vi "数据查询_仪器日志.vi"() -> ()   [LabVIEW 2016]
uses:
  <vilib>/Utility/miscctls.llb/LVPointTypeDef.ctl
  <vilib>/Utility/miscctls.llb/LVRowAndColumnUnsignedTypeDef.ctl
  <userlib>/_OpenG.lib/array/array.llb/Sort 2D Array (String)__ogtk.vi
panel:
  in  "页":i32 format="第%.0f页"
  in  "每页条数":i32=20
  in  "向后按钮":bool
  in  "向前按钮":bool
  in  "下拉列表":string(xcontrol)
  in  "导出":bool
  in  "查询":bool
  out "数据表":string[][](table)
  in  "结束日期":string="2050/01/01"
  in  "起始日期":string="2010/01/01"
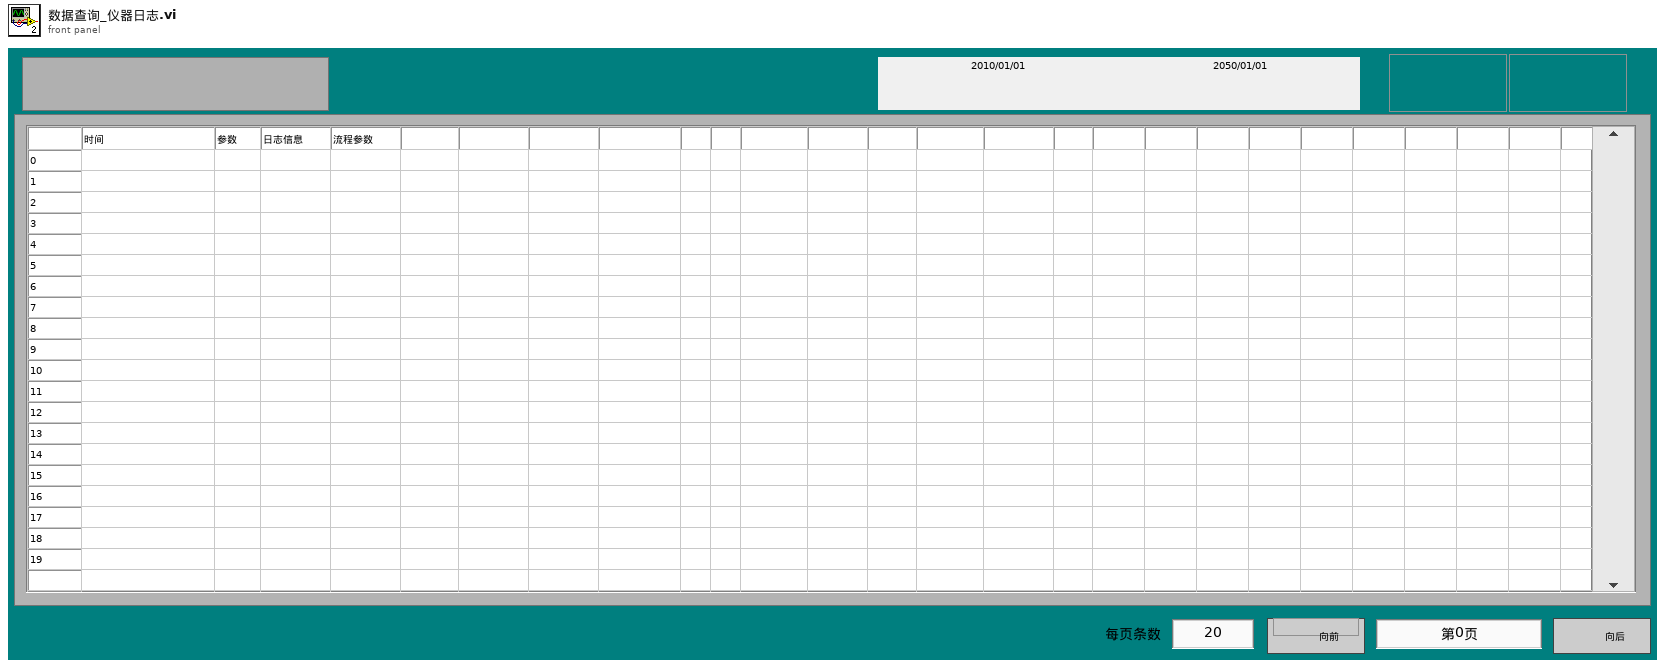
[diagram p1: front panel]
types:
  T1 = enum8{"Enabled", "Disabled", "Disabled and Grayed Out"}
  T2 = typedef "LVRowAndColumnUnsignedTypeDef.ctl" = cluster{"Row":u32, "Column":u32}
  T3 = typedef "LVPointTypeDef.ctl" = cluster{"Horizontal":i16, "Vertical":i16}
  T4 = typedef "LVDateTimeRec.ctl" = cluster{"秒数的小数部分":dbl, "秒":i32, "分":i32, "时":i32, "日":i32, "月":i32, "年":i32, "天数（周）":i32, "天数（年）":i32, "DST":i32}
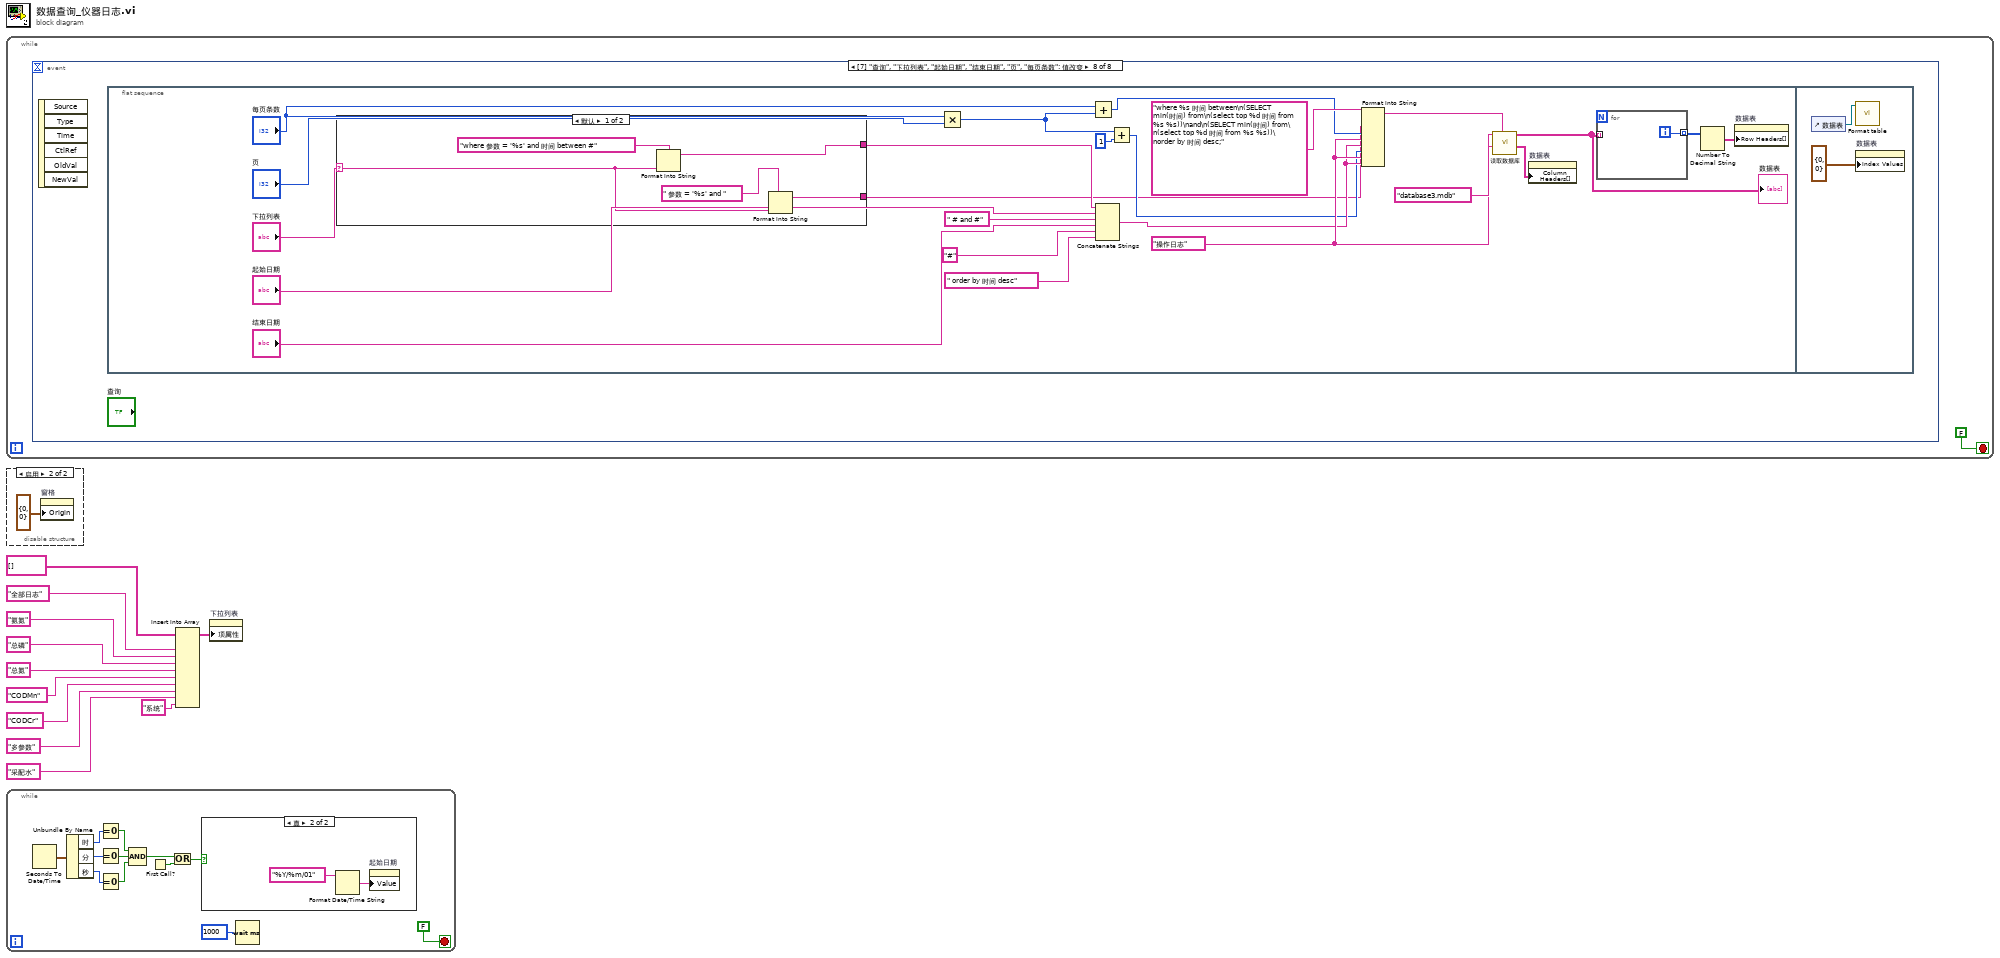
[diagram p0: block diagram]
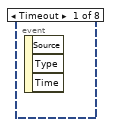
[diagram p3: hidden frame]
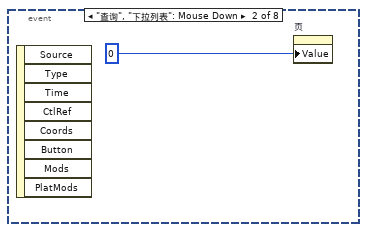
[diagram p4: hidden frame]
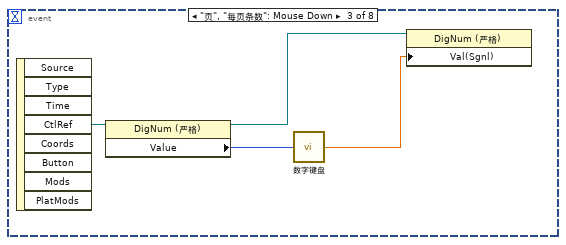
[diagram p5: hidden frame]
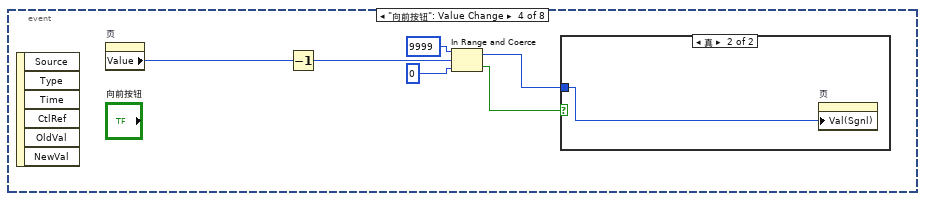
[diagram p6: hidden frame]
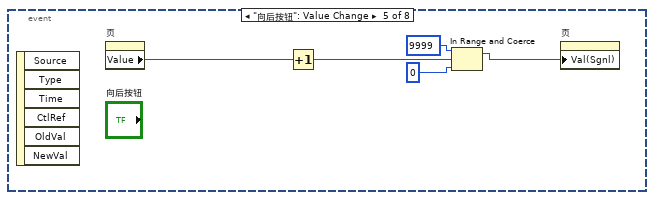
[diagram p8: hidden frame]
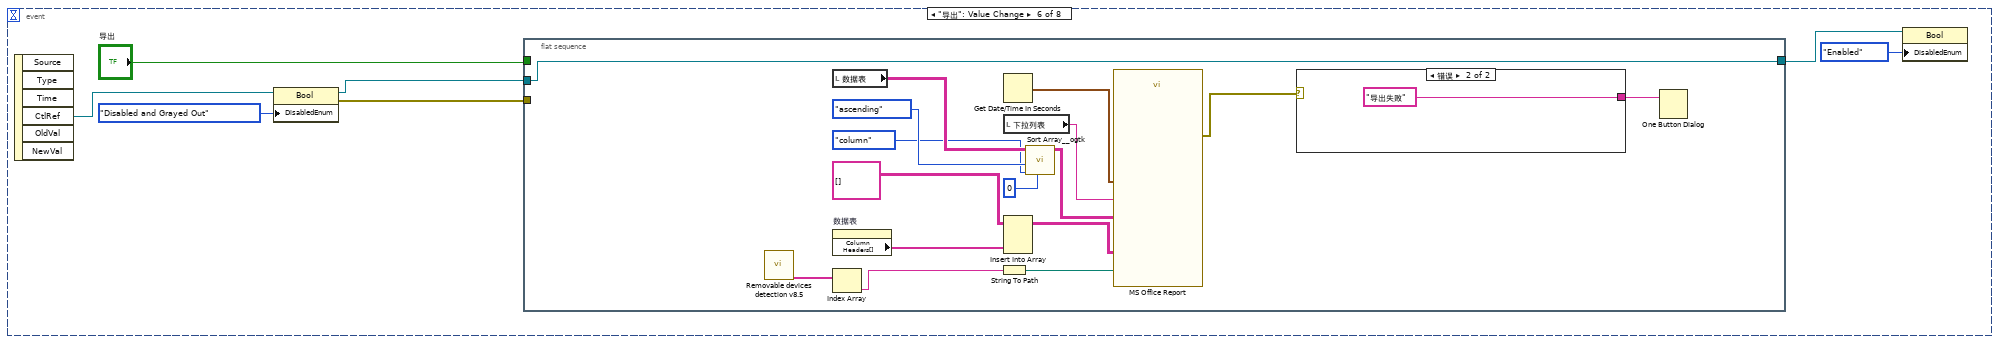
[diagram p9: hidden frame]
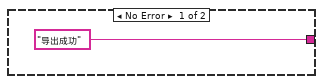
[diagram p10: hidden frame]
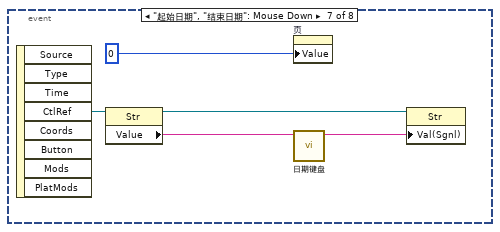
[diagram p11: hidden frame]
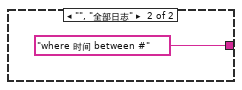
[diagram p12: hidden frame]
diagram:
  n1 = while {
    stop <- FALSE stop-if-true
    n2 = event shown="[7] \"查询\", \"下拉列表\", \"起始日期\", \"结束日期\", \"页\", \"每页条数\": 值改变" {
      selector: _ -> [_ _ _ _ _ _ _ _]
      dyn-events: _ -> [_ _ _ _ _ _ _ _]
      timeout: _ -> [_ _ _ _ _ _ _ _]
      event Timeout {
        n3 = event-data() -> ()  [unwired: 1 in, 3 out]
      }
      event "查询", "下拉列表": Mouse Down {
        n4 = event-data() -> ()  [unwired: 1 in, 8 out]
        n5 = property on="页" class="DigNum (严格)"("Value"=0 ("页")) -> ()  [unwired: 2 in, 2 out]
      }
      event "页", "每页条数": Mouse Down {
        n6 = event-data() -> ("CtlRef"=w17:refnum<vi>)  [unwired: 1 in, 7 out]
        n7 = property class="DigNum (严格)"(reference=w17) -> (reference out=w14:refnum<vi>, "Value"=w16:i32)  [unwired: 1 in, 1 out]
        n8 = call "数字键盘.vi"("OldNumber"=w16) -> ("NewNumber"=w15:sgl)
        n9 = property class="DigNum (严格)"(reference=w14, "Val(Sgnl)"=w15) -> ()  [unwired: 1 in, 2 out]
      }
      event "向前按钮": Value Change {
        n10 = event-data() -> ()  [unwired: 1 in, 6 out]
        n11 = property on="页" class="DigNum (严格)"() -> ("Value"=w23:i32)  [unwired: 2 in, 2 out]
        n12 = Decrement(x=w23) -> (x-1=w22:i32)
        n13 = In Range and Coerce(upper limit=9999 ("上限"), x=w22, lower limit=0 ("下限")) -> (coerced(x)=w19:i32, In Range?=w18:bool)
        n14 = case shown="真" w18 {
          tunnel: w19 -> [_ w24]
          frame False {
          }
          frame True {
            n15 = property on="页" class="DigNum (严格)"("Val(Sgnl)"=w24) -> ()  [unwired: 2 in, 2 out]
          }
        }
      }
      event "向后按钮": Value Change {
        n16 = event-data() -> ()  [unwired: 1 in, 6 out]
        n17 = property on="页" class="DigNum (严格)"() -> ("Value"=w29:i32)  [unwired: 2 in, 2 out]
        n18 = Increment(x=w29) -> (x+1=w28:i32)
        n19 = In Range and Coerce(upper limit=u32 9999 ("上限"), x=w28, lower limit=u32 0 ("下限")) -> (coerced(x)=w25:u32)  [unwired: 1 out]
        n20 = property on="页" class="DigNum (严格)"("Val(Sgnl)"=w25) -> ()  [unwired: 2 in, 2 out]
      }
      event "导出": Value Change {
        n21 = event-data() -> ("CtlRef"=w30:refnum<vi>)  [unwired: 1 in, 5 out]
        n22 = property class="Bool"(reference=w30, "DisabledEnum"=T1."Disabled and Grayed Out" ("禁用")) -> (reference out=w34:refnum<vi>, error out=w35:errorcluster)  [unwired: 1 in]
        n23 = flat-sequence {
          tunnel: w35 -> [_]
          tunnel: [w45] -> w33
          tunnel: w34 -> [w45]
          tunnel: "导出" -> [_]
          frame #0 {
            n24 = call "Removable devices detection v8.5.vi"() -> ("Removable"=w42:string[])  [unwired: 4 out]
            n25 = local read "数据表"() -> (w51:string[][])
            n26 = property on="数据表" class="Tbl (严格)"() -> ("Column Headers[]"=w37:string[])  [unwired: 2 in, 2 out]
            n27 = Index Array(array=w42) -> (element=w41:string)  [unwired: 1 in]
            n28 = String To Path(string=w41) -> (path=w40:path)
            n29 = Get Date/Time In Seconds() -> (seconds since 1Jan1904=w52:timestamp)
            n30 = local read "下拉列表"() -> (w46:string)
            n31 = Insert Into Array(array=string[][] [], new element=w37) -> (w38:string[][])  [unwired: 2 in]
            n32 = call-poly <userlib>:"Sort Array__ogtk.vi"("Column/Row to Sort By"=u32 0, "Sort By in"=enum16{"row", "column"}."column", "Order"=enum16{"ascending", "descending"}."ascending", "Array in"=w51) -> ("Sorted Array out"=w50:string[][])  [unwired: 4 in, 3 out]
            n33 = call "MS Office Report"("Path to Save Report"=w40, "导出日期"=w52, "监测参数"=w46, "数据输入"=w50, "字段定义"=w38) -> ("error out"=w44:errorcluster)  [unwired: 21 in, 1 out]
            n34 = case shown="错误" w44 {
              tunnel: ["导出成功" ("消息") "导出失败" ("消息")] -> w43
              frame No Error {
              }
              frame Error {
              }
            }
            n35 = One Button Dialog(message=w43) -> ()  [unwired: 1 in, 1 out]
          }
        }
        n36 = property class="Bool"(reference=w33, "DisabledEnum"=T1."Enabled" ("禁用")) -> ()  [unwired: 1 in, 2 out]
      }
      event "起始日期", "结束日期": Mouse Down {
        n37 = event-data() -> ("CtlRef"=w59:refnum<vi>)  [unwired: 1 in, 7 out]
        n38 = property class="Str"(reference=w59) -> (reference out=w57:refnum<vi>, "Value"=w58:string)  [unwired: 1 in, 1 out]
        n39 = property on="页" class="DigNum (严格)"("Value"=0 ("页")) -> ()  [unwired: 2 in, 2 out]
        n40 = call "日期键盘.vi"("原值"=w58) -> ("x+y"=w56:string)  [unwired: 10 in]
        n41 = property class="Str"(reference=w57, "Val(Sgnl)"=w56) -> ()  [unwired: 1 in, 2 out]
      }
      event "查询", "下拉列表", "起始日期", "结束日期", "页", "每页条数": Value Change {
        n42 = event-data() -> ()  [unwired: 1 in, 6 out]
        n43 = flat-sequence {
          frame #0 {
            w68 = "操作日志" ("组合框")
            n44 = case shown="默认" "下拉列表" {
              selector: "下拉列表" -> [w84 _]
              tunnel: [w87 "where 时间 between #" ("condition")] -> w72
              tunnel: [w83 _] -> w60
              frame Default {
                n45 = Format Into String(format string="where 参数 = '%s' and 时间 between #" ("condition"), w84) -> (resulting string=w87:string)  [unwired: 2 in, 1 out]
                n46 = Format Into String(format string=" 参数 = '%s' and " ("condition"), w84) -> (resulting string=w83:string)  [unwired: 2 in, 1 out]
              }
              frame "", "全部日志" {
              }
            }
            n47 = Multiply(x="每页条数", y="页") -> (x*y=w64:i32)
            n48 = Add(x="每页条数", y=w64) -> (x+y=w62:i32)
            n49 = Concatenate Strings(w72, "起始日期", " # and #" ("condition"), "结束日期", "#" ("condition"), " order by 时间 desc" ("字符串")) -> (w67:string)
            n50 = Add(x=w64, y=u32 1) -> (x+y=w61:u32)
            n51 = Format Into String(format string="where %s 时间 between\n(SELECT min(时间) from\n(select top %d 时间 from %s %s))\nand\n(SELECT min(时间) from\n(select top %d 时间 from %s %s))\norder by 时间 desc;" ("格式字符串"), w60, w62, w68, w67, w61, w68, w67) -> (resulting string=w69:string)  [unwired: 2 in, 1 out]
            n52 = call "读取数据库.vi"("condition"=w69, "database"="database3.mdb", "组合框"=w68) -> ("columns"=w78:string[], "表格"=w75:string[][])  [unwired: 5 in, 2 out]
            "数据表" <- w75
            n53 = property on="数据表" class="Tbl (严格)"("Column Headers[]"=w78) -> ()  [unwired: 2 in, 2 out]
            n54 = for {
              tunnel: w75 -> [_] mode=indexing
              tunnel: [w89] -> w74 mode=indexing
              i -> [w89]
            }
            n55 = Number To Decimal String(number=w74) -> (decimal integer string=w73:string[])  [unwired: 1 in]
            n56 = property on="数据表" class="Tbl (严格)"("Row Headers[]"=w73) -> ()  [unwired: 2 in, 2 out]
          }
          frame #1 {
            n57 = control-ref of="数据表"() -> (w90:refnum<vi>)
            n58 = call "Format table.vi"("Table输入"=w90) -> ()  [unwired: 11 in]
            n59 = property on="数据表" class="Tbl (严格)"("Index Values"=T2 {"Row"=0, "Column"=0} ("索引值")) -> ()  [unwired: 2 in, 2 out]
          }
        }
      }
    }
  }
  n60 = disable-structure shown="启用" {
    frame Disabled {
    }
    frame Enabled {
      n61 = property on="窗格" class="Pane"("Origin"=T3 {"Horizontal"=0, "Vertical"=0} ("原点")) -> ()  [unwired: 2 in, 2 out]
    }
  }
  n62 = while {
    stop <- FALSE stop-if-true
    n63 = Seconds To Date/Time() -> (date time rec=w104:T4)  [unwired: 2 in]
    n64 = Unbundle By Name(w104) -> ("时"=w103:i32, "分"=w102:i32, "秒"=w101:i32)
    n65 = Equal To 0?(x=w103) -> (x = 0?=w100:bool)
    n66 = Equal To 0?(x=w102) -> (x = 0?=w99:bool)
    n67 = Equal To 0?(x=w101) -> (x = 0?=w98:bool)
    n68 = Compound Arithmetic op=AND ("复合运算")(w100, w99, w98) -> (w95:bool)
    n69 = First Call?() -> (First Call?: T/F=w93:bool)
    n70 = Or(x=w95, y=w93) -> (x .or. y?=w94:bool)
    n71 = case shown="真" w94 {
      frame False {
      }
      frame True {
        n72 = Format Date/Time String(time format string (%c)="%Y/%m/01" ("时间格式字符串(%c)")) -> (date/time string=w105:string)  [unwired: 2 in]
        n73 = property on="起始日期" class="Str"("Value"=w105) -> ()  [unwired: 2 in, 2 out]
      }
    }
    n74 = Wait (ms)(milliseconds to wait=u32 1000 ("等待时间（毫秒）")) -> ()  [unwired: 1 out]
  }
  n75 = Insert Into Array(array=string[] [], new element #1="全部日志" ("新元素/子数组"), new element #2="氨氮" ("新元素/子数组"), new element #3="总磷" ("新元素/子数组"), new element #4="总氮" ("新元素/子数组"), new element #5="CODMn" ("新元素/子数组"), new element #6="CODCr" ("新元素/子数组"), new element #7="多参数" ("新元素/子数组"), new element #8="采配水" ("新元素/子数组"), new element #9="系统" ("新元素/子数组")) -> (w1:string[])  [unwired: 1 in]
  n76 = property on="下拉列表" class="下拉列表 (严格)"("项属性"=w1) -> ()  [unwired: 2 in, 2 out]
